vi "AccelerationBrakeDetect.vi"(5 "油门1输入":dbl format="%#_16g", 6 "油门2输入":dbl format="%#_16g", 7 "刹车输入":dbl format="%#_16g") -> (0 "油门1":dbl format="%#_16g", 1 "油门2":dbl format="%#_16g", 2 "刹车":dbl format="%#_616g", 3 "上次运行有故障？":bool, 4 "Implausibility":bool=TRUE)   [LabVIEW 2013]
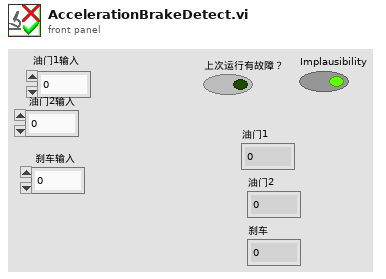
[diagram p1: front panel]
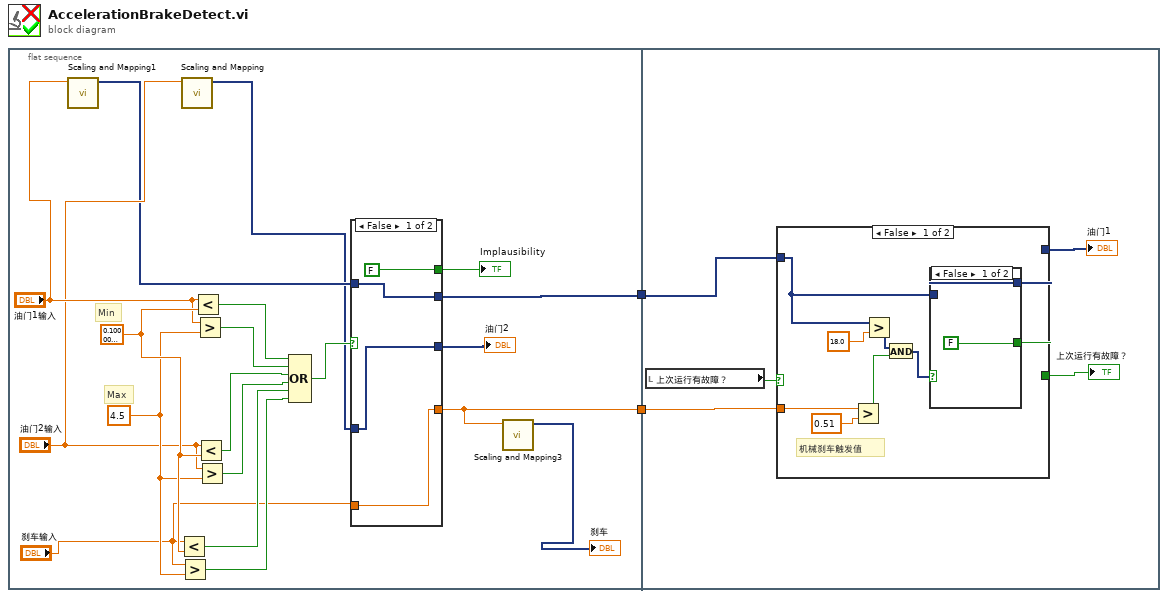
[diagram p0: block diagram]
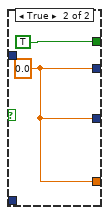
[diagram p2: hidden frame]
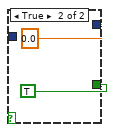
[diagram p3: hidden frame]
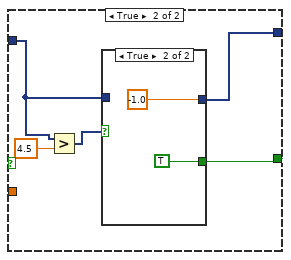
[diagram p4: hidden frame]
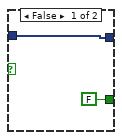
[diagram p5: hidden frame]
diagram:
  n1 = flat-sequence {
    tunnel: [w21] -> w2
    tunnel: [w5] -> w1
    tunnel: w2 -> [w32]
    tunnel: w1 -> [w30]
    frame #0 {
      w12 = sgl 4.5 ("y")
      w13 = sgl 0.1 ("y")
      # "Min"
      # "Max"
      n2 = call "Scaling and Mapping1"("Signals"="油门1输入") -> ("Scaled Signals"=w6:dynamicdata)  [unwired: 9 in, 1 out]
      n3 = Less?(x="刹车输入", y=w13) -> (x < y?=w15:bool)
      n4 = Greater?(x="刹车输入", y=w12) -> (0:w14:bool)
      n5 = call "Scaling and Mapping"("Signals"="油门2输入") -> ("Scaled Signals"=w3:dynamicdata)  [unwired: 9 in, 1 out]
      n6 = Less?(x="油门1输入", y=w13) -> (x < y?=w19:bool)
      n7 = Greater?(x="油门1输入", y=w12) -> (0:w18:bool)
      n8 = Less?(x="油门2输入", y=w13) -> (x < y?=w17:bool)
      n9 = Greater?(x="油门2输入", y=w12) -> (0:w16:bool)
      n10 = Compound Arithmetic op=OR(w19, w18, w17, w16, w15, w14) -> (w20:bool)
      n11 = case shown="False" w20 {
        tunnel: [w25 w27] -> w21
        tunnel: [w22 w27] -> w11
        tunnel: [w23 w27] -> w5
        tunnel: w6 -> [w25 _]
        tunnel: w3 -> [w22 _]
        tunnel: "刹车输入" -> [w23 _]
        tunnel: [FALSE TRUE] -> w9
        frame False {
        }
        frame True {
          w27 = 0.0
        }
      }
      "Implausibility" <- w9
      "油门2" <- w11
      n12 = call "Scaling and Mapping3"("Signals"=w5) -> ("Scaled Signals"=→"刹车":dynamicdata)  [unwired: 9 in, 1 out]
    }
    frame #1 {
      n13 = local read "上次运行有故障？"() -> (w29:bool)
      n14 = case shown="False" w29 {
        tunnel: w32 -> [w34 w46]
        tunnel: [w37 w48] -> w31
        tunnel: w30 -> [w36 _]
        tunnel: [w35 w47] -> w28
        frame False {
          # "机械刹车触发值"
          n15 = Greater?(x=w36, y=0.51) -> (0:w39:bool)
          n16 = Greater?(x=w34, y=18.0) -> (0:w40:dynamicdata)
          n17 = And(x=w40, y=w39) -> (x .and. y?=w38:dynamicdata)
          n18 = case shown="False" w38 {
            tunnel: w34 -> [w43 _]
            tunnel: [w43 0.0 ("油门1")] -> w37
            tunnel: [FALSE ("上次运行有故障？") TRUE ("上次运行有故障？")] -> w35
            frame False {
            }
            frame True {
            }
          }
        }
        frame True {
          n19 = Greater?(x=w46, y=4.5) -> (0:w49:dynamicdata)
          n20 = case shown="True" w49 {
            tunnel: [w52 -1.0 ("油门1")] -> w48
            tunnel: w46 -> [w52 _]
            tunnel: [FALSE ("上次运行有故障？") TRUE ("上次运行有故障？")] -> w47
            frame False {
            }
            frame True {
            }
          }
        }
      }
      "油门1" <- w31
      "上次运行有故障？" <- w28
    }
  }
